vi "executeMP.vi"(8 "error in (no error)":errorcluster, 10 "Subsystems":T1, 11 "Parser in":refnum<class "CommandCreator.lvclass">) -> (0 "error out":errorcluster, 2 "command":string, 3 "Parser out":refnum<class "CommandCreator.lvclass">)   [LabVIEW 2016, in "CommandCreator.lvclass"]
uses:
  CommandCreator.lvclass
  AlCS/Subsystems.ctl
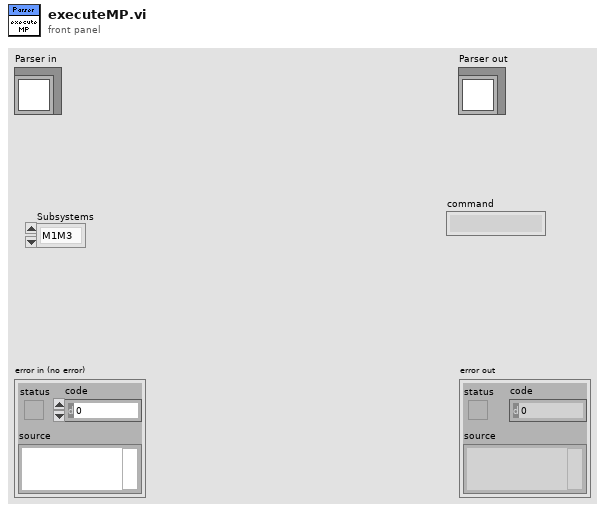
[diagram p1: front panel]
types:
  T1 = typedef "Subsystems.ctl" = enum16{"M1M3", "Camera", "M2"}
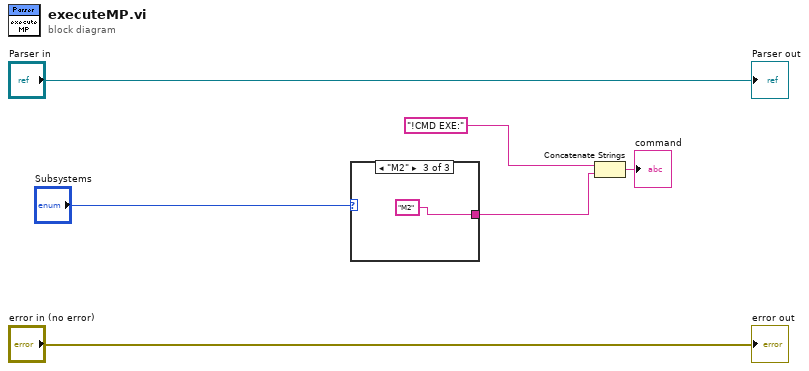
[diagram p0: block diagram]
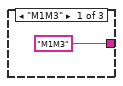
[diagram p2: hidden frame]
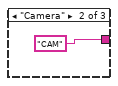
[diagram p3: hidden frame]
diagram:
  n1 = case shown="\"M2\"" "Subsystems" {
    tunnel: ["M1M3" "CAM" "M2"] -> w2
    frame "M1M3" {
    }
    frame "Camera" {
    }
    frame "M2" {
    }
  }
  n2 = Concatenate Strings("!CMD EXE:", w2) -> (→"command":string)
  "error out" <- "error in (no error)"
  "Parser out" <- "Parser in"
